vi "lsl push chunk d.vi"(8 "error in (no error)":errorcluster, 9 "data_elements":i64, 10 "data":dbl[][](array[numeric]), 11 "outlet":T1) -> (0 "error out":errorcluster, 2 "function return":i32)   [LabVIEW 2019, in "Lab Streaming Layer.lvlib"]
doc: "extern LIBLSL_C_API int32_t lsl_push_chunk_d(lsl_outlet out, const double *data, unsigned long data_elements);"
uses:
  Lab Streaming Layer.lvlib
  Custom Controls/lsl_outlet.ctl
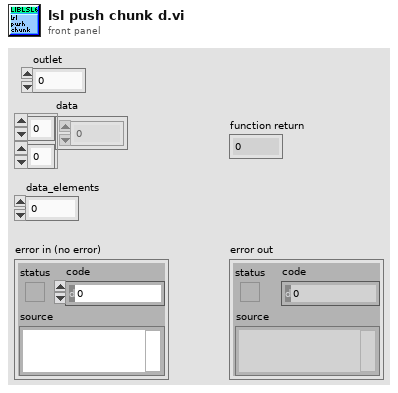
[diagram p1: front panel]
types:
  T1 = typedef "Lab Streaming Layer.lvlib/lsl_outlet.ctl" = u64
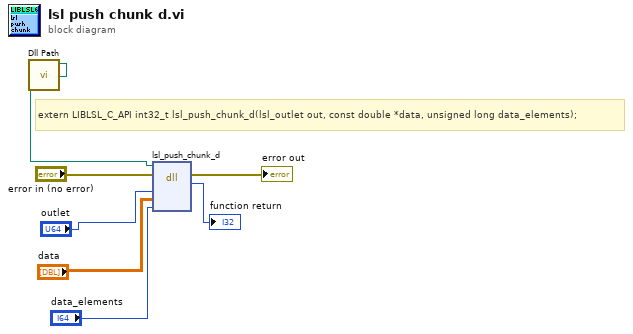
[diagram p0: block diagram]
diagram:
  # "extern LIBLSL_C_API int32_t lsl_push_chunk_d(lsl_outlet out, const double *data, unsigned long data_elements);"
  n1 = call "Dll Path.vi"() -> ("Dll path"=w1:path)  [unwired: 11 in]
  n2 = dll-call lib="E:/LabStreamingLayer/liblsl-LabVIEW-master/liblsl-LabVIEW-master/lsl.dll" fn="lsl_push_chunk_d"(path in=w1, error in="error in (no error)", "out"="outlet", "data"="data", "data_elements"="data_elements") -> (error out=→"error out":errorcluster, "return type"=→"function return":i32)  [unwired: 4 in, 1 out]
